vi "DisplayConsole_DataCluster.vi"(8 "error in (no error)":errorcluster) -> (0 "error out":errorcluster, 3 "DataCluster":T1)   [LabVIEW 2013, in "DisplayConsoleLib.lvlib"]
uses:
  DisplayConsoleLib.lvlib
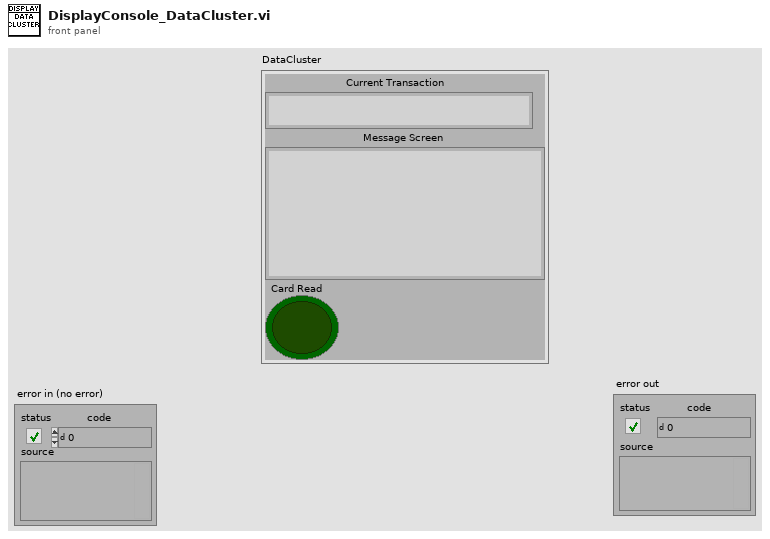
[diagram p1: front panel]
types:
  T1 = cluster{"Current Transaction":string, "Message Screen":string, "Card Read":bool}
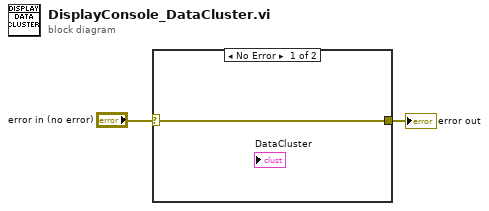
[diagram p0: block diagram]
diagram:
  n1 = case shown="No Error" "error in (no error)" {
    selector: "error in (no error)" -> [w3 w4]
    tunnel: [w3 w4] -> w1
    frame No Error {
    }
    frame Error {
    }
  }
  "error out" <- w1
